vi "OTP_Bundle.vi"() -> ()   [LabVIEW 2020, in "Test Framework.lvclass"]
uses:
  Test Framework.lvclass
panel:
  in  "Test Framework.lvclass":refnum<class "Test Framework.lvclass">
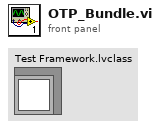
[diagram p1: front panel]
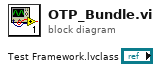
[diagram p0: block diagram]
diagram:
